vi "Configure Trigger (Edge).vi"(0 "VISA resource name":refnum<visa-resource-name>, 5 "Trigger Source (1: Channel 1)":u16(ring)=1 items=["Channel 1"=1, "Channel 2"=2, "Channel 3"=3, "Channel 4"=4, "External"=5, "External 5"=6, "AC Line"=7], 7 "Trigger Slope (0: Positive)":u16(ring) items=["Positive", "Negative", "Alternation"], 9 "Trigger Level (0.0 V)":dbl, 11 "error in (no error)":errorcluster, 12 "Trigger Modifier (0: Auto)":u16(ring) items=["Auto", "Normal", "Single"]) -> (4 "VISA resource name out":refnum<visa-resource-name>, 15 "error out":errorcluster)   [LabVIEW 2010, in "Agilent DSO1000 Series.lvlib"]
doc: "Configures edge trigger settings. An edge trigger occurs when the trigger signal passes through the voltage threshold that you specify with the <B>Trigger Level</B> control and has the slope that you specify with the <B>Trigger Slope</B> control."
uses:
  <instrlib>/Agilent DSO1000 Series/Agilent DSO1000 Series.lvlib
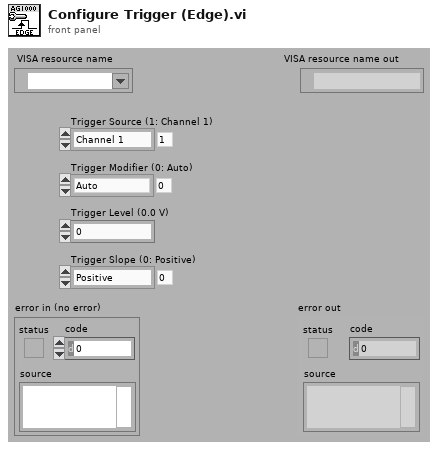
[diagram p1: front panel]
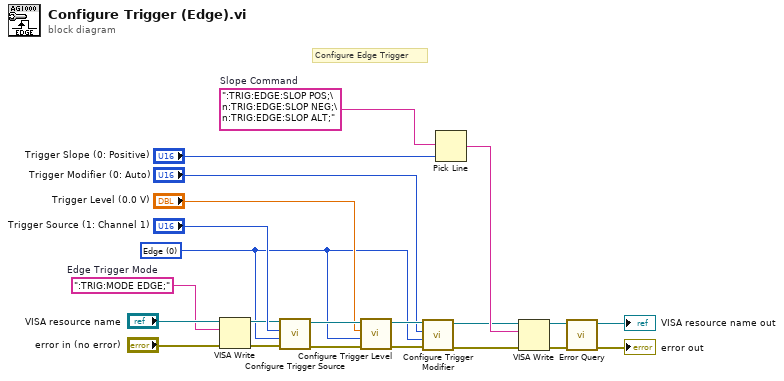
[diagram p0: block diagram]
diagram:
  w1 = u16 0 items=["Edge", "Pulse", "TV", "Pattern"] ("Trigger Type")
  w18 = ":TRIG:EDGE:SLOP POS;\n:TRIG:EDGE:SLOP NEG;\n:TRIG:EDGE:SLOP ALT;"  # Slope Command
  w14 = ":TRIG:MODE EDGE;"  # Edge Trigger Mode
  # "Configure Edge Trigger"
  n1 = VISA Write(VISA resource name="VISA resource name", write buffer=w14, error in (no error)="error in (no error)") -> (VISA resource name out=w12:refnum<visa-resource-name>, error out=w11:errorcluster)  [unwired: 1 out]
  n2 = call <instrlib>:"Configure Trigger Source.vi"("error in (no error)"=w11, "Trigger Type"=w1, "Trigger Source (1: Channel 1)"="Trigger Source (1: Channel 1)", "VISA resource name"=w12) -> ("error out"=w10:errorcluster, "VISA resource name out"=w9:refnum<visa-resource-name>)  [unwired: 6 in]
  n3 = call <instrlib>:"Configure Trigger Level.vi"("error in (no error)"=w10, "Trigger Type"=w1, "Trigger Level (0.0 V)"="Trigger Level (0.0 V)", "VISA resource name"=w9) -> ("error out"=w7:errorcluster, "VISA resource name out"=w6:refnum<visa-resource-name>)  [unwired: 6 in]
  n4 = call <instrlib>:"Configure Trigger Modifier.vi"("error in (no error)"=w7, "Trigger Type"=w1, "Trigger Modifier (0: Auto)"="Trigger Modifier (0: Auto)", "VISA resource name"=w6) -> ("error out"=w2:errorcluster, "VISA resource name out"=w3:refnum<visa-resource-name>)  [unwired: 6 in]
  n5 = Pick Line(multi-line string=w18, line index="Trigger Slope (0: Positive)") -> (output string=w4:string)  [unwired: 1 in]
  n6 = VISA Write(VISA resource name=w3, write buffer=w4, error in (no error)=w2) -> (VISA resource name out=w20:refnum<visa-resource-name>, error out=w19:errorcluster)  [unwired: 1 out]
  n7 = call <instrlib>:"Error Query.vi"("error in (no error)"=w19, "VISA resource name"=w20) -> ("error out"=→"error out":errorcluster, "VISA resource name out"=→"VISA resource name out":refnum<visa-resource-name>)  [unwired: 6 in, 2 out]
